vi "Measurement UI.vi"() -> ()   [LabVIEW 2022 SP3, in "Calibrate Acoustic Output Level UI.lvlib"]
uses:
  Calibrate Acoustic Output Level UI.lvlib
  <vilib>/Utility/miscctls.llb/LVPointTypeDef.ctl
panel:
  out "time domain":waveform(dbl)(graph)
  out "wfm - data":dbl[](array[numeric])
  out "wfm - dt":dbl
  in  "output channel":string="PXI1Slot4/ai0"
  in  "ref mic channel":string="PXI1Slot4/ai0"
  in  "Configuration tab":enum32{"Measurement"}(tab)
  out "output voltage ratio":dbl caption="Output voltage ratio" format="%#.3f Pa/Vpk"
  in  "number of steps":dbl=3.39 caption="Number of steps" format="%#.3f"
  in  "Output Channel":tag="PXI1Slot2/ao0" caption="Channel"
  in  "target value (dB)":dbl=94.0 caption="Target level" format="%#_3f dBSPL"
  in  "Ref Mic Channel":tag="PXI1Slot2/ai0" caption="Channel"
  in  "ref mic sensitivity (mV/Pa)":dbl=50.0 caption="Sensitivity" format="%#.6f mV/Pa"
  in  "frequency":dbl=1000.0 caption="Frequency" format="%#_6pHz"
  in  "start amplitude (Vpk)":dbl=3.39 caption="Start amplitude" format="%#.3f Vpk"
  in  "stop amplitude (Vpk)":dbl=3.39 caption="Stop amplitude" format="%#.3f Vpk"
  # "Output"
  # "Reference Microphone"
  # "Results"
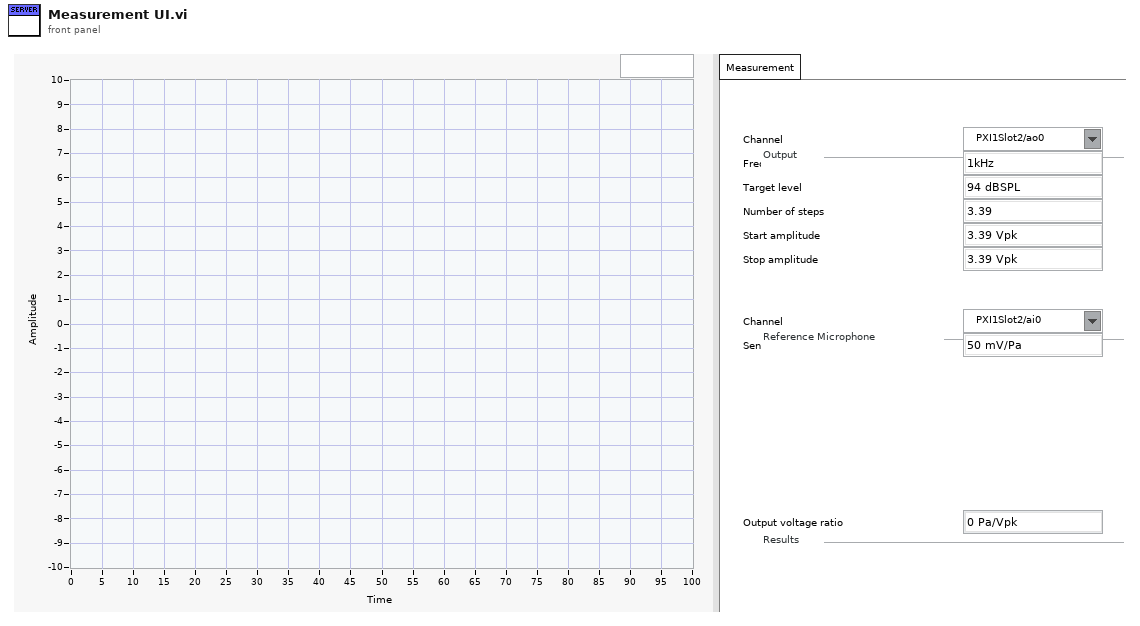
[diagram p1: front panel]
types:
  T1 = typedef "LVPointTypeDef.ctl" = cluster{"Horizontal":i16, "Vertical":i16}
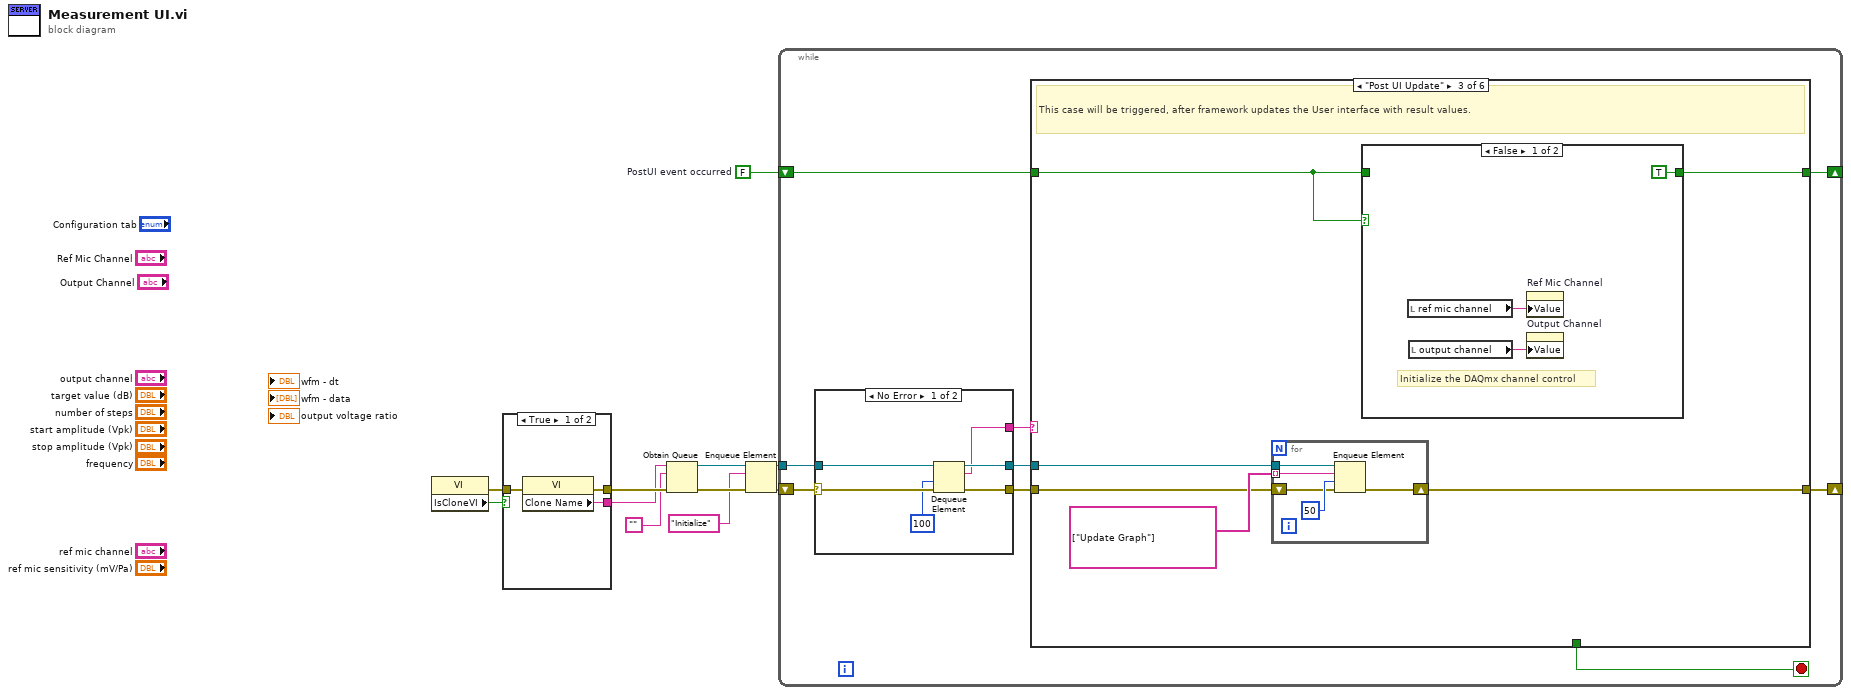
[diagram p0: block diagram]
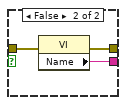
[diagram p2: hidden frame]
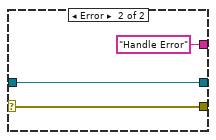
[diagram p3: hidden frame]
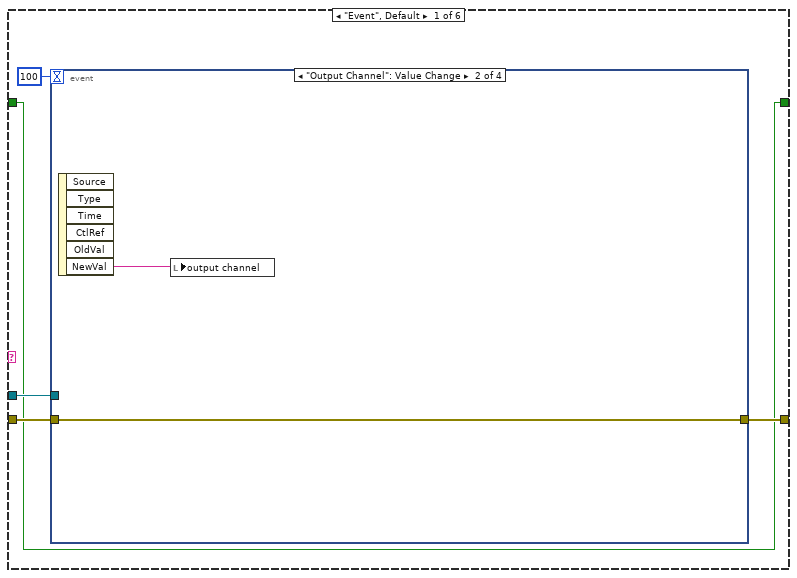
[diagram p4: hidden frame]
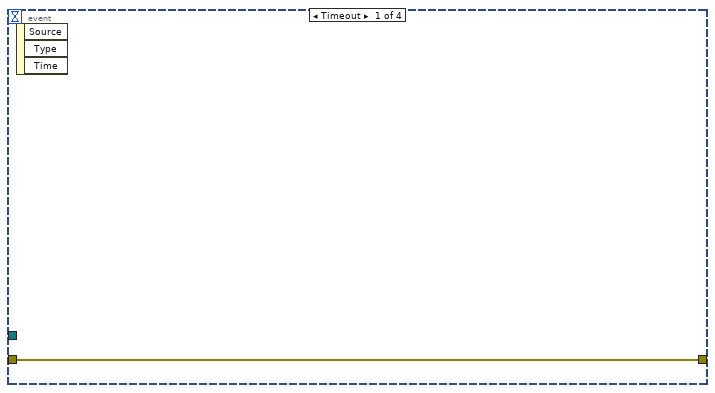
[diagram p5: hidden frame]
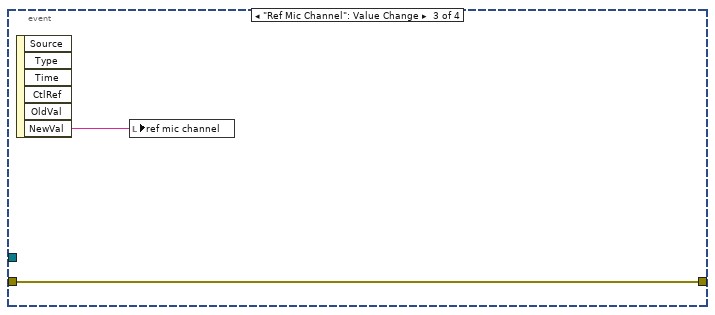
[diagram p6: hidden frame]
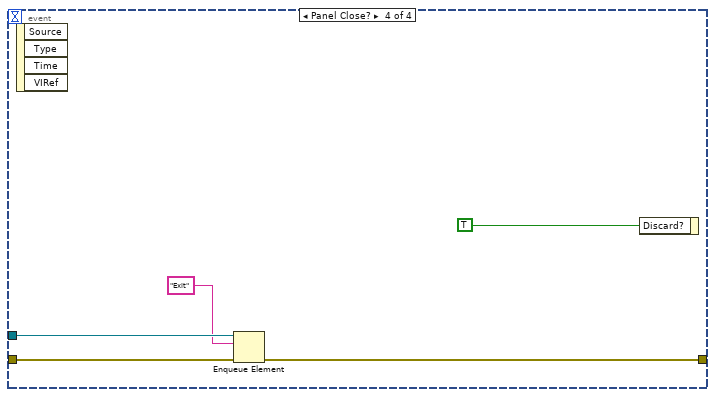
[diagram p7: hidden frame]
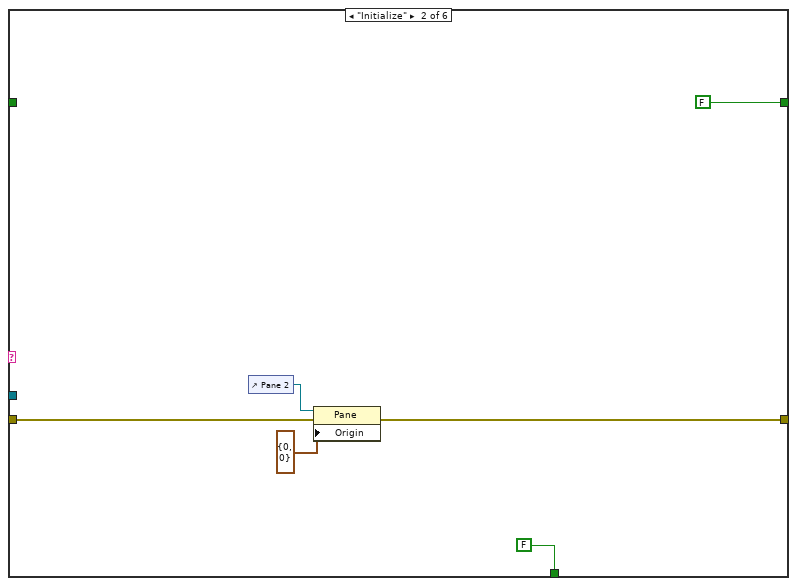
[diagram p8: hidden frame]
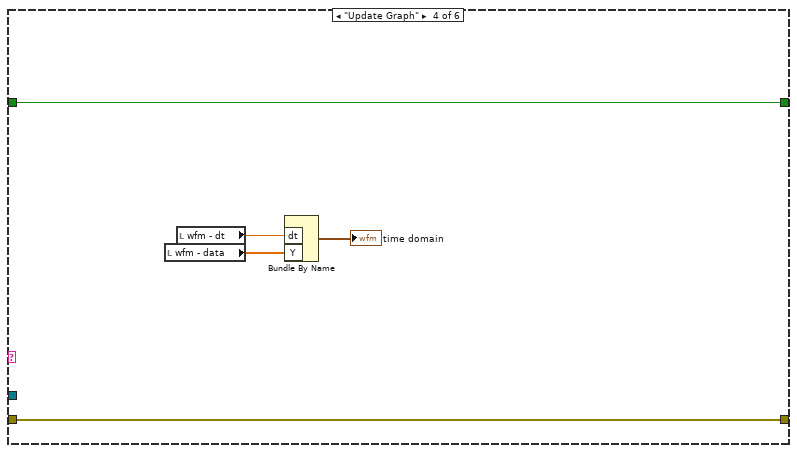
[diagram p10: hidden frame]
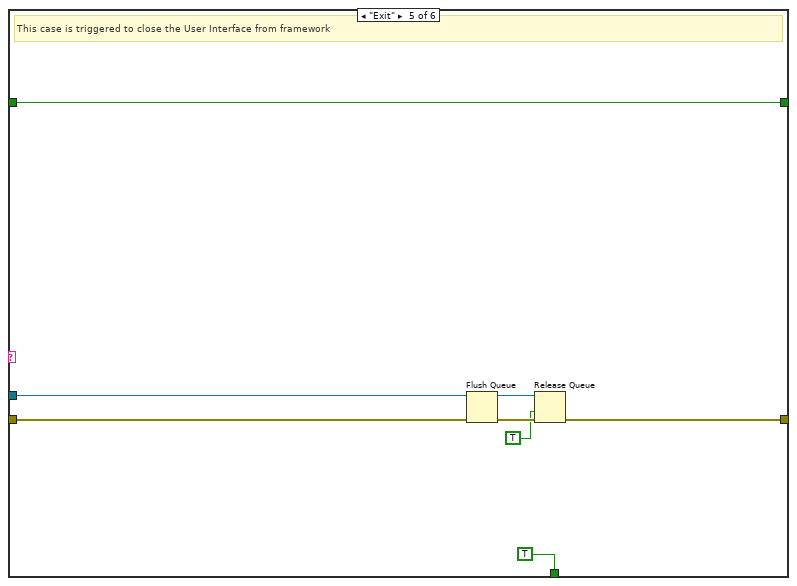
[diagram p11: hidden frame]
diagram:
  w1 = FALSE  # PostUI event occurred
  n1 = property class="VI"() -> (error out=w2:errorcluster, "IsCloneVI"=w3:bool)  [unwired: 2 in, 1 out]
  n2 = case shown="True" w3 {
    tunnel: [w14 w17] -> w11
    tunnel: [w13 w16] -> w10
    tunnel: w2 -> [w12 w15]
    frame True {
      n3 = property class="VI"(error in=w12) -> (error out=w14:errorcluster, "Clone Name"=w13:string)  [unwired: 1 in, 1 out]
    }
    frame False {
      n4 = property class="VI"(error in=w15) -> (error out=w17:errorcluster, "Name"=w16:string)  [unwired: 1 in, 1 out]
    }
  }
  n5 = Obtain Queue(name (unnamed)=w10, element data type="", error in (no error)=w11) -> (queue out=w7:refnum<queue>, error out=w9:errorcluster)  [unwired: 2 in, 1 out]
  n6 = Enqueue Element(queue=w7, element="Initialize", error in (no error)=w9) -> (queue out=w6:refnum<queue>, error out=w8:errorcluster)  [unwired: 1 in, 1 out]
  n7 = while {
    shift-right: [w21] -> _
    shift-left: w8 -> [w26]
    tunnel: w6 -> [w24]
    shift-right: [w18] -> _
    shift-left: w1 -> [w19]
    stop <- w20 stop-if-true
    n8 = case shown="No Error" w26 {
      selector: w26 -> [w32 w35]
      tunnel: [w31 w35] -> w25
      tunnel: w24 -> [w30 w34]
      tunnel: [w29 w34] -> w23
      tunnel: [w28 "Handle Error"] -> w22
      frame No Error {
        n9 = Dequeue Element(queue=w30, timeout in ms (-1)=100, error in (no error)=w32) -> (queue out=w29:refnum<queue>, element=w28:string, error out=w31:errorcluster)  [unwired: 1 out]
      }
      frame Error {
      }
    }
    n10 = case shown="\"Post UI Update\"" w22 {
      tunnel: w25 -> [w39 w54 w59 w73 w84 w86]
      tunnel: w23 -> [w37 _ w58 _ w82 _]
      tunnel: [w40 w53 w57 w73 w79 w86] -> w21
      tunnel: [_ FALSE _ _ TRUE _] -> w20
      tunnel: w19 -> [w36 _ w62 w72 w77 w85]
      tunnel: [w36 FALSE ("PostUI event occurred") w61 w72 w77 w85] -> w18
      frame "Event", Default {
        n11 = event shown="[1] \"Output Channel\": Value Change" {
          selector: _ -> [_ _ _ _]
          dyn-events: _ -> [_ _ _ _]
          timeout: 100 -> [_ _ _ _]
          tunnel: [w41 w42 w44 w48] -> w40
          tunnel: w39 -> [w41 w42 w44 w49]
          tunnel: w37 -> [_ _ _ w47]
          event Timeout {
            n12 = event-data() -> ()  [unwired: 1 in, 3 out]
          }
          event "Output Channel": Value Change {
            n13 = event-data() -> ("NewVal"=w43:tag)  [unwired: 1 in, 5 out]
            n14 = local write "output channel"(w43) -> ()
          }
          event "Ref Mic Channel": Value Change {
            n15 = event-data() -> ("NewVal"=w45:tag)  [unwired: 1 in, 5 out]
            n16 = local write "ref mic channel"(w45) -> ()
          }
          event Panel Close? {
            n17 = event-data() -> ()  [unwired: 1 in, 4 out]
            n18 = Enqueue Element(queue=w47, element="Exit", error in (no error)=w49) -> (error out=w48:errorcluster)  [unwired: 1 in, 2 out]
            n19 = event-data("Discard?"=TRUE) -> ()  [unwired: 1 in, 1 out]
          }
        }
      }
      frame "Initialize" {
        n20 = control-ref of="Pane 2"() -> (w52:refnum<vi>)
        n21 = property class="Pane"(reference=w52, error in=w54, "Origin"=T1 {"Horizontal"=0, "Vertical"=0}) -> (error out=w53:errorcluster)  [unwired: 1 out]
      }
      frame "Post UI Update" {
        # "This case will be triggered, after framework updates the User interface with result values."
        n22 = for {
          tunnel: w58 -> [w65]
          shift-right: [w64] -> w57
          shift-left: w59 -> [w66]
          tunnel: string[] ["Update Graph"] -> [w63] mode=indexing
          n23 = Enqueue Element(queue=w65, element=w63, timeout in ms (-1)=50, error in (no error)=w66) -> (error out=w64:errorcluster)  [unwired: 2 out]
        }
        n24 = case shown="False" w62 {
          tunnel: w62 -> [_ w71]
          tunnel: [TRUE ("PostUI event occurred") w71] -> w61
          frame False {
            # "Initialize the DAQmx channel control"
            n25 = local read "ref mic channel"() -> (w68:string)
            n26 = local read "output channel"() -> (w69:string)
            n27 = property on="Ref Mic Channel" class="DAQmxName"("Value"=w68) -> ()  [unwired: 2 in, 2 out]
            n28 = property on="Output Channel" class="DAQmxName"("Value"=w69) -> ()  [unwired: 2 in, 2 out]
          }
          frame True {
          }
        }
      }
      frame "Update Graph" {
        n29 = local read "wfm - data"() -> (w76:dbl[])
        n30 = local read "wfm - dt"() -> (w75:dbl)
        n31 = Bundle By Name("dt"=w75, "Y"=w76) -> (→"time domain":waveform(dbl))  [unwired: 1 in]
      }
      frame "Exit" {
        # "This case is triggered to close the User Interface from framework"
        n32 = Flush Queue(queue=w82, error in (no error)=w84) -> (queue out=w81:refnum<queue>, error out=w80:errorcluster)  [unwired: 1 out]
        n33 = Release Queue(queue=w81, force destroy? (F)=TRUE, error in (no error)=w80) -> (error out=w79:errorcluster)  [unwired: 2 out]
      }
      frame "Handle Error" {
      }
    }
  }
